vi "Get Sentence Parts.vi"(8 "error in (no error)":errorcluster, 11 "sentence":string) -> (0 "error out":errorcluster, 1 "valid sentence?":bool, 3 "sentence data":string[](array[string]))   [LabVIEW 2017, in "NMEA API.lvlib"]
doc: "Returns an array of values contained in an NMEA <B>sentence</B>."
uses:
  <vilib>/robotics/Protocols/NMEA/NMEA API.lvlib
  <vilib>/regexp/Match Regular Expression.xnode
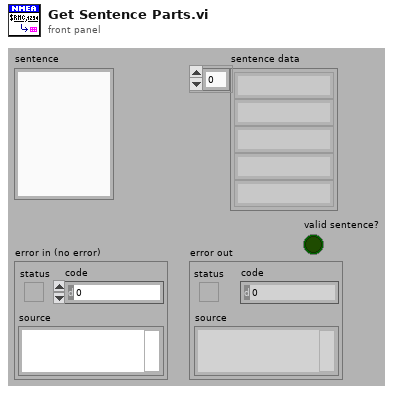
[diagram p1: front panel]
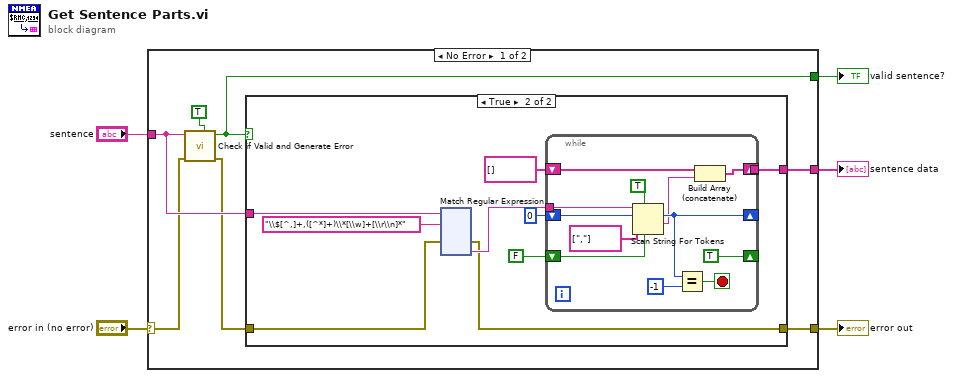
[diagram p0: block diagram]
diagram:
  n1 = case shown="No Error" "error in (no error)" {
    selector: "error in (no error)" -> [w9 w148]
    tunnel: [w12 w148] -> w4
    tunnel: [w11 _] -> w3
    tunnel: "sentence" -> [w10 _]
    tunnel: [w7 _] -> w1
    frame No Error {
      n2 = call <vilib>:"Check if Valid and Generate Error.vi"("generate error if invalid (F)"=TRUE, "error in (no error)"=w9, "sentence"=w10) -> ("error out"=w8:errorcluster, "valid sentence"=w7:bool)  [unwired: 7 in]
      n3 = case shown="True" w7 {
        tunnel: [w13 w16] -> w12
        tunnel: w8 -> [w13 w20]
        tunnel: [_ w14] -> w11
        tunnel: w10 -> [_ w22]
        frame False {
          # "Invalid sentence"
        }
        frame True {
          n4 = xnode "Match Regular Expression"("input string"=w22, "regular expression"="\\$[^,]+,([^*]+)\\*[\\w]+[\\r\\n]*", "error in"=w20) -> ("error out"=w16:errorcluster, "submatch 1"=w19:string)  [unwired: 1 in, 6 out]
          n5 = while {
            tunnel: w19 -> [w31]
            shift-right: [w30] -> _
            shift-left: 0 ("offset past token") -> [w32]
            shift-right: [TRUE] -> _
            shift-left: FALSE -> [w28]
            shift-right: [w23] -> w14
            shift-left: string[] [] -> [w24]
            tunnel: [w23] -> _
            stop <- w29 stop-if-true
            n6 = Scan String For Tokens(4:w28, 5:TRUE ("allow empty tokens? (F)"), 6:string[] [","] ("delimiters (\\s,\\t,\\r,\\n)"), 8:w32, 9:w31) -> (1:w25:string, 2:w30:i32)  [unwired: 3 out]
            n7 = Equal?(x=w30, y=-1) -> (x = y?=w29:bool)
            n8 = Build Array (concatenate)(w24, w25) -> (w23:string[])
          }
        }
      }
    }
    frame Error {
    }
  }
  "error out" <- w4
  "sentence data" <- w3
  "valid sentence?" <- w1
